vi "Run VI Method.vi"() -> ()   [LabVIEW 2020]
panel:
  in  "stop":bool
  out "iterations":i32
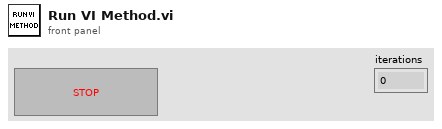
[diagram p1: front panel]
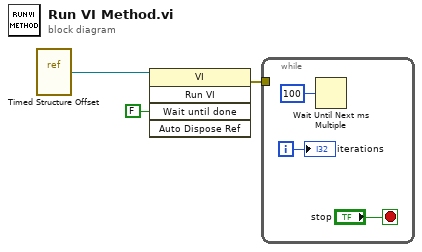
[diagram p0: block diagram]
diagram:
  n1 = vi-ref "Timed Structure Offset.vi"() -> (w3:refnum<vi>)
  n2 = invoke class="VI" method="Run VI"(reference=w3, "Wait until done"=FALSE ("Wait Until Done")) -> (error out=w2:errorcluster)  [unwired: 3 in, 4 out]
  n3 = while {
    tunnel: w2 -> [_]
    i -> [w6]
    stop <- "stop" stop-if-true
    n4 = Wait Until Next ms Multiple(millisecond multiple=u32 100) -> ()  [unwired: 1 out]
    "iterations" <- w6
  }
